vi "searchItem.vi"(0 "reference in":refnum<class "Project Panels.lvclass">=refnum, 11 "error in (no error)":errorcluster) -> (4 "reference out":refnum<class "Project Panels.lvclass">, 6 "Sheet out":T1=enum."storage", 10 "indexElements":i32[](array[numeric]), 15 "error out":errorcluster)   [LabVIEW 2014, in "Project Panels.lvclass"]
uses:
  Project Panels.lvclass
  SYS/Items Controller_llb/storageSheets.ctl
  SYS/Items Controller_llb/itemsColumn.ctl
  deviceState.ctl
  SYS/Items Controller_llb/Items Controller.lvclass
panel:
  in  "Item Column:":T2
  in  "Stop Button":bool
  out "Status bar":string="Fill in the control and press Sarch Item button....."
  in  "Search Item":bool
  in  "Item:":string
  in  "Sheet:":T1
  out "title":string="Searching Item Panel"
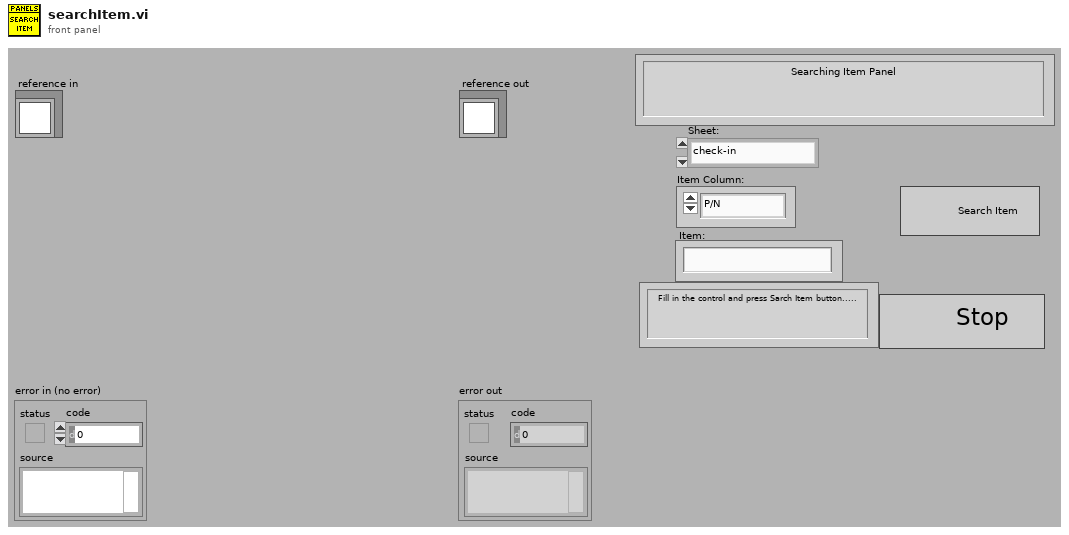
[diagram p1: front panel]
types:
  T1 = typedef "Items Controller.lvclass/storageSheets.ctl" = enum16{"check-in", "check-out", "storage"}
  T2 = typedef "Items Controller.lvclass/itemsColumn.ctl" = enum16{"P/N", "S/N", "Description"}
  T3 = typedef "Project Panels.lvclass/deviceState.ctl" = enum16{"check", "initiate", "waitEvent", "dataFromPDF", "getDetails", "save", "close", "stop"}
  T4 = typedef "Project Panels.lvclass/ObjectAttributesRef.ctl" = refnum<data-value>
  T5 = typedef "Project Panels.lvclass/ObjectAttributes.ctl" = cluster{"MyAttribute":dbl, "device_controller_ref":refnum<class "Devices Controller.lvclass">, "file_controller_ref":refnum<class "File Controller.lvclass">, "item_controller_ref":refnum<class "Items Controller.lvclass">, "item_tables":cluster{"checkIN":string[][], "checkOUT":string[][], "storage":string[][]}, "quickbook_table":cluster{"notes":string[][]}, "notification_controller_ref":refnum<class "Notification Controller.lvclass">, "partstracking_controller_ref":refnum<class "PartsTracking Controller.lvclass">, "product_tables":cluster{"k4b2":string[][], "fitmate":string[][], "RMR":string[][], "CPET":string[][], "BP":string[][], "PP":string[][], "k5":string[][], "bb-pft":string[][]}, "rowsColour":u32[]}
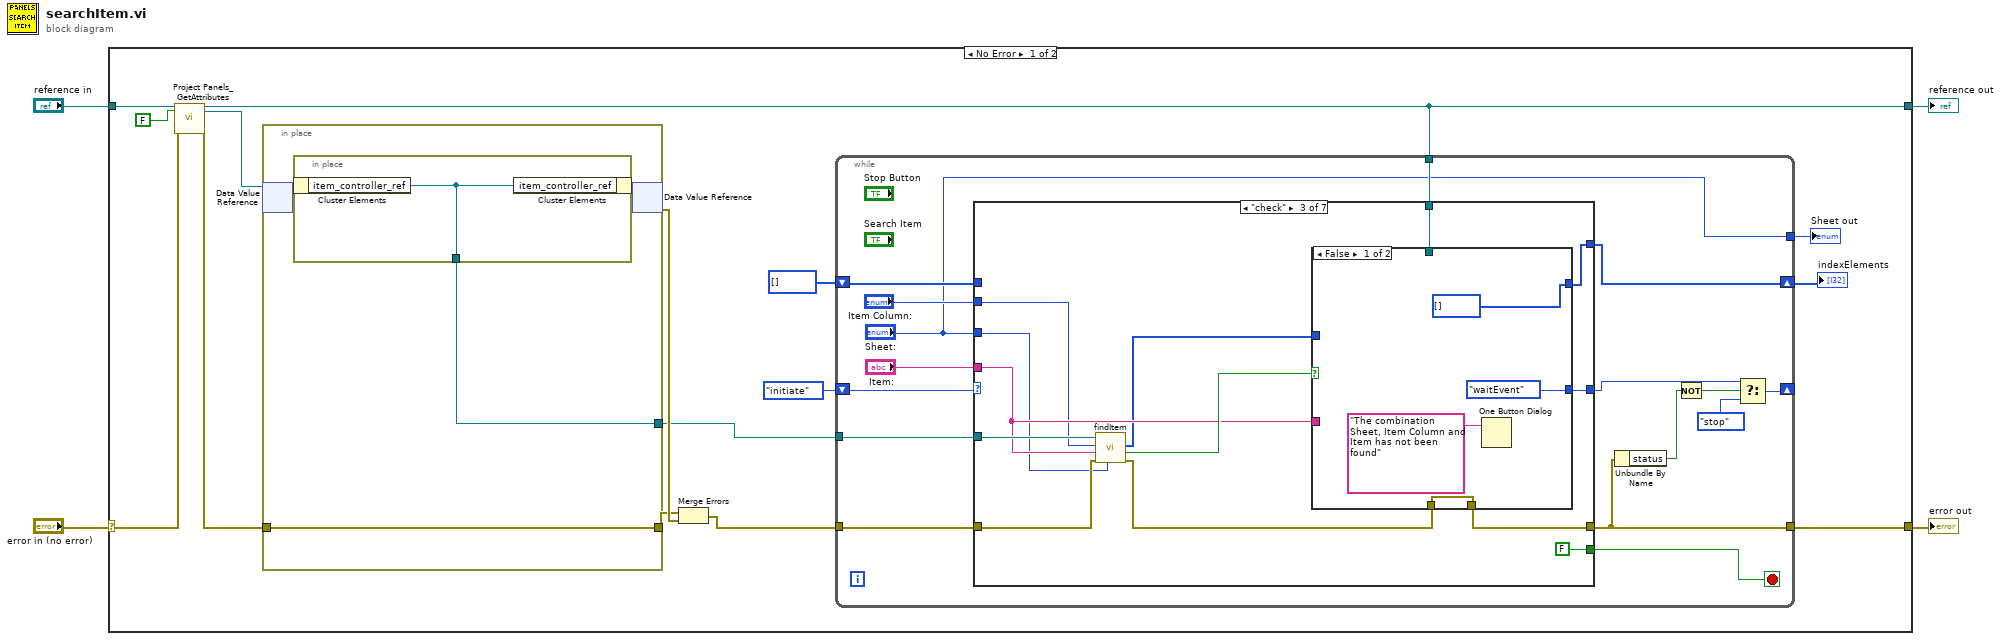
[diagram p0: block diagram]
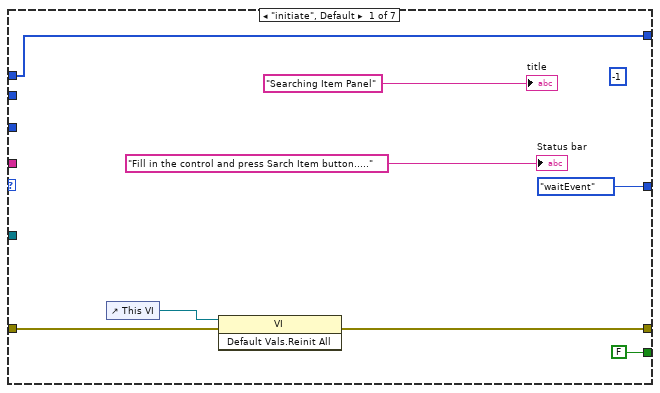
[diagram p2: hidden frame]
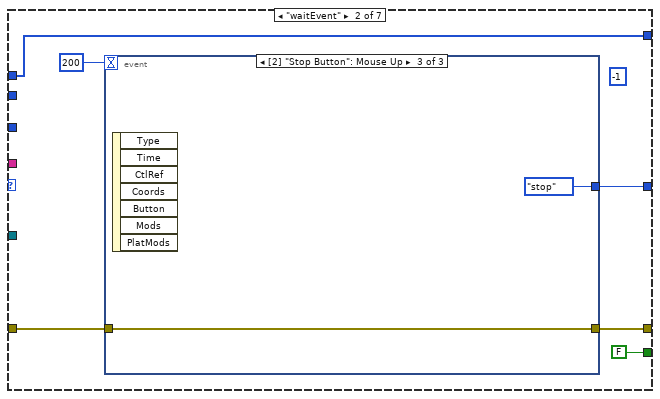
[diagram p3: hidden frame]
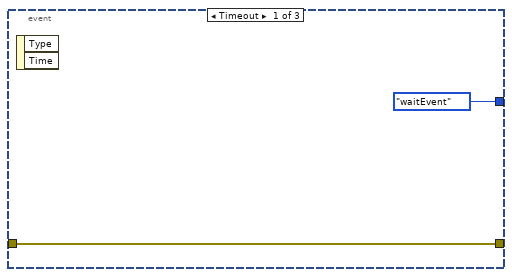
[diagram p4: hidden frame]
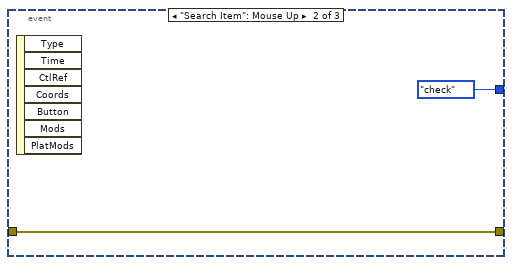
[diagram p5: hidden frame]
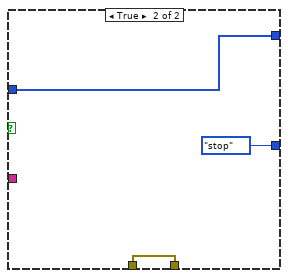
[diagram p6: hidden frame]
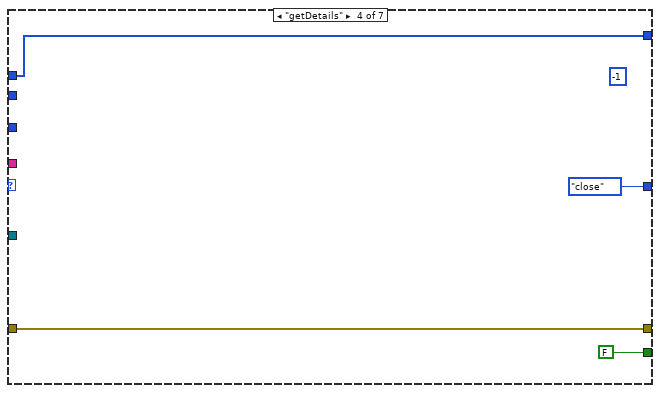
[diagram p7: hidden frame]
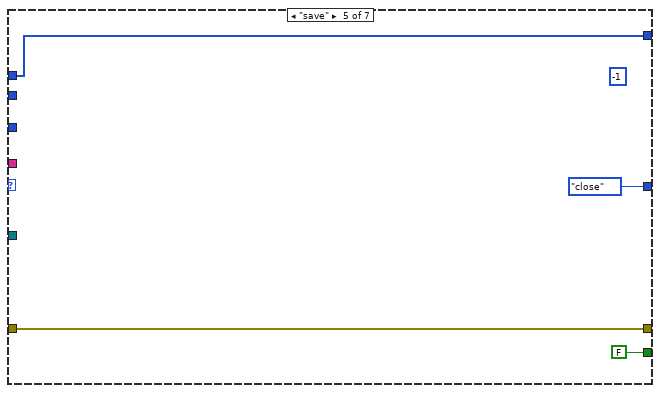
[diagram p8: hidden frame]
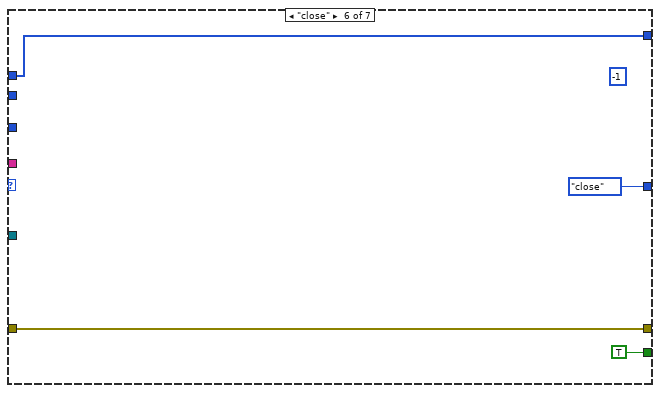
[diagram p9: hidden frame]
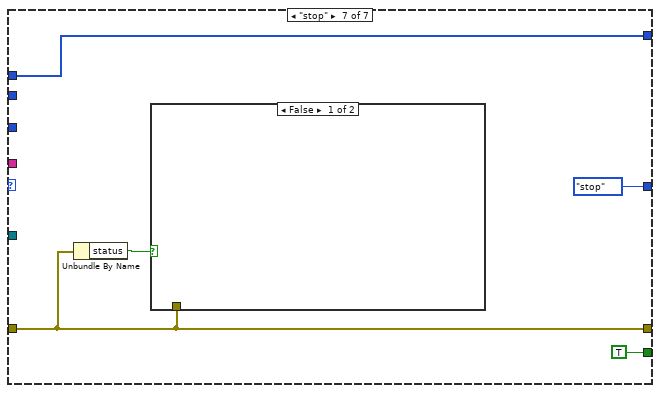
[diagram p10: hidden frame]
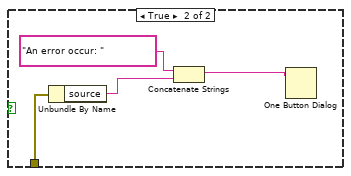
[diagram p11: hidden frame]
diagram:
  n1 = case shown="No Error" "error in (no error)" {
    selector: "error in (no error)" -> [w15 w103]
    tunnel: [w12 w103] -> w3
    tunnel: [w10 w102] -> w1
    tunnel: "reference in" -> [w17 w102]
    frame No Error {
      n2 = call "Project Panels_GetAttributes.vi"("reference in"=w17, "return data? (T)"=FALSE, "error in (no error)"=w15) -> ("reference out"=w10:refnum<class "Project Panels.lvclass">, "attributes ref"=w13:T4, "error out"=w14:errorcluster)  [unwired: 13 in, 1 out]
      n3 = in-place {
        in-place-border: w14 -> [w98]
        in-place-border: [w98] -> w18
        in-place-border: [w97] -> w8
        n4 = in-place-dvr #1(w13) -> (w99:T5)  [unwired: 1 out]
        n5 = in-place {
          in-place-border: [w101] -> w97
          n6 = in-place-cluster #2(w99) -> ("item_controller_ref"=w101:refnum<class "Items Controller.lvclass">)
          n7 = in-place-cluster #2("item_controller_ref"=w101) -> (w100:T5)
        }
        n8 = in-place-dvr #1(w100) -> (w19:errorcluster)  [unwired: 1 out]
      }
      n9 = Merge Errors(w18, w19) -> (w9:errorcluster)
      n10 = while {
        tunnel: w9 -> [w35]
        tunnel: [w31] -> w12
        shift-right: [w32] -> _
        shift-left: deviceState."initiate" ("state") -> [w34]
        tunnel: w10 -> [w26]
        tunnel: w8 -> [w24]
        shift-right: [w20] -> w5
        shift-left: i32[] [] -> [w23]
        tunnel: ["Sheet:"] -> w7
        stop <- w25 stop-if-true
        n11 = case shown="\"check\"" w34 {
          tunnel: w35 -> [w38 w49 w64 w78 w82 w86 w89]
          tunnel: [w37 w48 w66 w78 w82 w86 w89] -> w31
          tunnel: [deviceState."waitEvent" ("state") w46 w68 deviceState."close" ("f") deviceState."close" ("f") deviceState."close" ("f") deviceState."stop" ("f")] -> w33
          tunnel: "Sheet:" -> [_ _ w59 _ _ _ _]
          tunnel: "Item:" -> [_ _ w60 _ _ _ _]
          tunnel: w26 -> [_ _ w67 _ _ _ _]
          tunnel: [FALSE FALSE FALSE FALSE FALSE TRUE TRUE] -> w25
          tunnel: w24 -> [_ _ w62 _ _ _ _]
          tunnel: w23 -> [w36 w44 _ w76 w80 w84 w88]
          tunnel: "Item Column:" -> [_ _ w58 _ _ _ _]
          tunnel: [w36 w44 w56 w76 w80 w84 w88] -> w20
          frame "initiate", Default {
            (unwired) -1 ("indexElement")
            n12 = control-ref of="This VI"() -> (w39:refnum<vi>)
            n13 = invoke class="VI" method="Default Vals.Reinit All"(reference=w39, error in=w38) -> (error out=w37:errorcluster)  [unwired: 1 in, 2 out]
            "title" <- "Searching Item Panel" ("title")
            "Status bar" <- "Fill in the control and press Sarch Item button....." ("Status bar")
          }
          frame "waitEvent" {
            (unwired) -1 ("indexElement")
            n14 = event shown="[2] \"Stop Button\": Mouse Up" {
              selector: _ -> [_ _ _]
              dyn-events: _ -> [_ _ _]
              timeout: 200 -> [_ _ _]
              tunnel: w49 -> [w51 w53 w54]
              tunnel: [w51 w53 w54] -> w48
              tunnel: [deviceState."waitEvent" ("f") deviceState."check" ("f") deviceState."stop" ("f")] -> w46
              event Timeout {
                n15 = event-data() -> ()  [unwired: 1 in, 2 out]
              }
              event "Search Item": Mouse Up {
                n16 = event-data() -> ()  [unwired: 1 in, 7 out]
              }
              event "Stop Button": Mouse Up {
                n17 = event-data() -> ()  [unwired: 1 in, 7 out]
              }
            }
          }
          frame "check" {
            n18 = call "findItem.vi"("storageSheets"=w59, "error in (no error)"=w64, "item"=w60, "itemColumn"=w58, "reference in"=w62) -> ("error out"=w63:errorcluster, "found!"=w61:bool, "indexElements"=w57:i32[])  [unwired: 3 in, 1 out]
            n19 = case shown="False" w61 {
              tunnel: [deviceState."waitEvent" ("state") deviceState."stop" ("state")] -> w68
              tunnel: w67 -> [_ _]
              tunnel: w63 -> [w70 w74]
              tunnel: [w70 w74] -> w66
              tunnel: w60 -> [_ _]
              tunnel: w57 -> [_ w73]
              tunnel: [i32[] [] w73] -> w56
              frame False {
                n20 = One Button Dialog(message="The combination Sheet, Item Column and Item has not been found") -> ()  [unwired: 1 in, 1 out]
              }
              frame True {
              }
            }
          }
          frame "getDetails" {
            (unwired) -1 ("indexElement")
          }
          frame "save" {
            (unwired) -1 ("indexElement")
          }
          frame "close" {
            (unwired) -1 ("indexElement")
          }
          frame "stop" {
            n21 = Unbundle By Name(w89) -> ("status"=w90:bool)
            n22 = case shown="False" w90 {
              tunnel: w89 -> [_ w93]
              frame False {
              }
              frame True {
                n23 = Unbundle By Name(w93) -> ("source"=w94:string)
                n24 = Concatenate Strings("An error occur: " ("message"), w94) -> (w95:string)
                n25 = One Button Dialog(message=w95) -> ()  [unwired: 1 in, 1 out]
              }
            }
          }
        }
        n26 = Unbundle By Name(w31) -> ("status"=w30:bool)
        n27 = Not(x=w30) -> (.not. x?=w29:bool)
        n28 = Select(t=w33, s=w29, f=deviceState."stop") -> (s? t:f=w32:T3)
      }
      "Sheet out" <- w7
      "indexElements" <- w5
    }
    frame Error {
    }
  }
  "error out" <- w3
  "reference out" <- w1
